vi "Ex-2 FPGA.vi"() -> ()   [LabVIEW 2014]
uses:
  <vilib>/rvi/Emulation/niFpgaGetClockAttributes.vi
  <vilib>/rvi/Emulation/niFpgaSctlEmulationGetInTimedLoop.vi
  <vilib>/rvi/Emulation/niFpgaEmulationReportErrorSimple.vi
  <vilib>/rvi/Emulation/niFpgaProcessEmulError.vi
  <vilib>/rvi/interface/RandomDataEmulation/niFpgaRandomDataHandleErrors.vi
  <vilib>/rvi/Emulation/niFpgaCriticalErrorInLSC.vi
  <vilib>/rvi/DataTransferAndStorage/Container/XNode/niFpgaContainer.xnode
  <vilib>/rvi/interface/RandomDataEmulation/nirviRandomDataFpgaReadWriteTemplate.vi
panel:
  in  "Data to Host":u64
  out "FPGA Error":errorcluster
  out "Finished":bool
  in  "stop":bool
  out "Module Underflow":bool
  out "Acq Loop Ticks":u32
  out "DMA FIFO Full":bool
  out "Chan Count":bool
  out "First Read":bool
  in  "Number of Channels":i32=4
  in  "Acquisition Type":enum16{"Finite Samples", "Continuous Samples"}(ring)
  in  "Samps per Chan [Finite]":i32=5120
  in  "Chan Scale Array":sgl[](array[numeric])=[0.0, 0.0, 0.0, 0.0, 0.0, 0.0, 0.0, 0.0, 0.0, 0.0, 0.0, 0.0, 0.0, 0.0, 0.0, 0.0, 0.0, 0.0, 0.0, 0.0, 0.0, 0.0, 0.0, 0.0, 0.0, 0.0, 0.0, 0.0, 0.0, 0.0, 0.0, 0.0, 0.0, 0.0, 0.0, 0.0, 0.0, 0.0, 0.0, 0.0]
  out "oclk mult":u32
  out "oclk div":u32
  out "oclk freq":u32
  in  "data rate (S/s)":u32
  # "Array size fixed at 40\nelements but may be \nexpanded if needed"
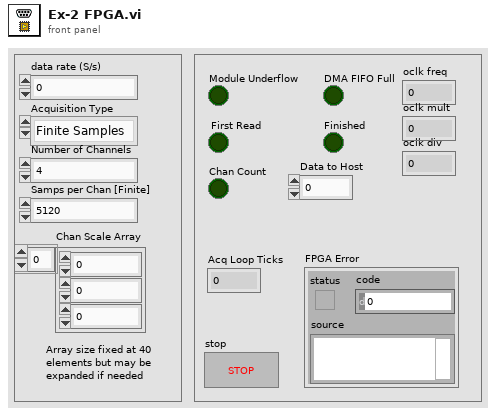
[diagram p1: front panel]
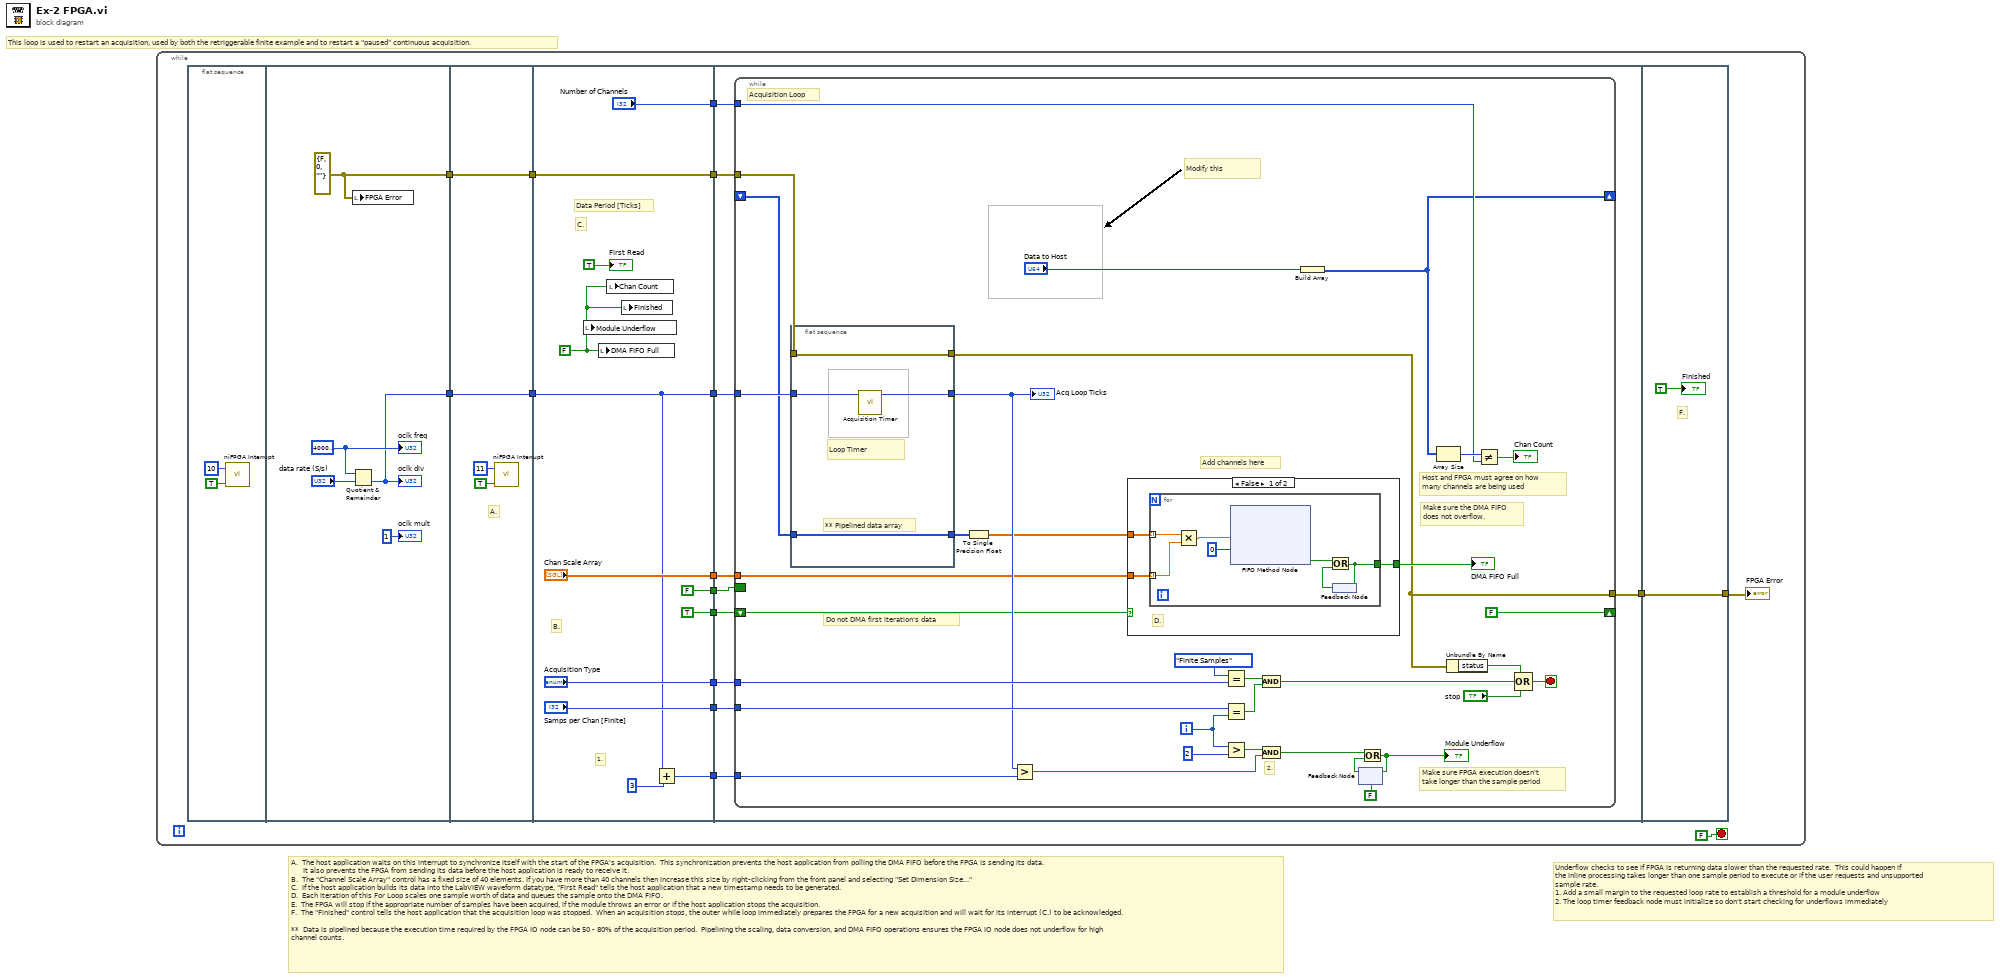
[diagram p0: block diagram]
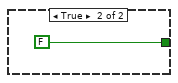
[diagram p2: hidden frame]
diagram:
  # "Underflow checks to see if FPGA is returning data slower than the requested rate.  This could happen if\nthe inline processing takes longer than one sample period to execute or if the user requests and unsupported\nsample rate.\n1. Add a small margin to the requested loop rate to establish a threshold for a module underflow \n2. The loop timer feedback node must initialize so don't start checking for underflows immediately"
  # "A.  The host application waits on this interrupt to synchronize itself with the start of the FPGA's acquisition.  This synchronization prevents the host application from polling the DMA FIFO before the FPGA is sending its data.\n      It also prevents the FPGA from sending its data before the host application is ready to receive it.\nB.  The \"Channel Scale Array\" control has a fixed size of 40 elements. If you have more than 40 channels then increase this size by right-clicking from the front panel and selecting \"Set Dimension Size...\"\nC.  If the host application builds its data into the LabVIEW waveform datatype, \"First Read\" tells the host application that a new timestamp needs to be generated.\nD.  Each iteration of this For Loop scales one sample worth of data and queues the sample onto the DMA FIFO.  \nE.  The FPGA will stop if the appropriate number of samples have been acquired, if the module throws an error or if the host application stops the acquisition.  \nF.  The \"Finished\" control tells the host application that the acquisition loop was stopped.  When an acquisition stops, the outer while loop immediately prepares the FPGA for a new acquisition and will wait for its interrupt (C.) to be acknowledged. \n\n**  Data is pipelined because the execution time required by the FPGA IO node can be 50 - 80% of the acquisition period.  Pipelining the scaling, data conversion, and DMA FIFO operations ensures the FPGA IO node does not underflow for high\nchannel counts."
  # "This loop is used to restart an acquisition, used by both the retriggerable finite example and to restart a \"paused\" continuous acquisition."
  n1 = while {
    stop <- FALSE stop-if-true
    n2 = flat-sequence {
      tunnel: [w20] -> w9
      tunnel: [w19] -> w5
      tunnel: w9 -> [w25]
      tunnel: [w25] -> w8
      tunnel: [w24] -> w6
      tunnel: w5 -> [w24]
      tunnel: ["Number of Channels"] -> w16
      tunnel: ["Chan Scale Array"] -> w15
      tunnel: ["Acquisition Type"] -> w14
      tunnel: ["Samps per Chan [Finite]"] -> w13
      tunnel: [w29] -> w12
      tunnel: [w33] -> w11
      tunnel: [TRUE] -> w10
      tunnel: w8 -> [w30]
      tunnel: [w30] -> w7
      tunnel: w6 -> [w29]
      tunnel: [FALSE] -> w4
      tunnel: w16 -> [w49]
      tunnel: w15 -> [w46]
      tunnel: w14 -> [w45]
      tunnel: w13 -> [w44]
      tunnel: w12 -> [w47]
      tunnel: w11 -> [w43]
      tunnel: w10 -> [w42]
      tunnel: w7 -> [w48]
      tunnel: w4 -> [w41]
      tunnel: [w40] -> w2
      tunnel: [w99] -> w1
      tunnel: w2 -> [w99]
      frame #0 {
        n3 = call <vilib>:"niFPGA Interrupt.vi"("Wait Until Cleared (F)"=TRUE ("Wait Until Cleared"), "IRQ Number (0)"=u8 10 ("IRQ Number")) -> ()  [unwired: 1 in]
      }
      frame #1 {
        w20 = errorcluster {"status"=FALSE, "code"=0, "source"=""} ("FPGA Error")
        w21 = u32 40000000 ("oclk freq")
        n4 = Quotient & Remainder(x=w21, y="data rate (S/s)") -> (floor(x/y)=w19:u32)  [unwired: 1 out]
        "oclk div" <- w19
        n5 = local write "FPGA Error"(w20) -> ()
        "oclk mult" <- u32 1 ("oclk mult")
        "oclk freq" <- w21
      }
      frame #2 {
        # "A."
        n6 = call <vilib>:"niFPGA Interrupt.vi"("Wait Until Cleared (F)"=TRUE ("Wait Until Cleared"), "IRQ Number (0)"=u8 11 ("IRQ Number")) -> ()  [unwired: 1 in]
      }
      frame #3 {
        w38 = FALSE ("Module Underflow")
        # "Data Period [Ticks]"
        # "1."
        # "C."
        # "B."
        n7 = local write "Module Underflow"(w38) -> ()
        n8 = local write "DMA FIFO Full"(w38) -> ()
        n9 = local write "Chan Count"(w38) -> ()
        n10 = local write "Finished"(w38) -> ()
        n11 = Add(x=w29, y=u32 3) -> (x+y=w33:u32)
        "First Read" <- TRUE ("First Read")
      }
      frame #4 {
        n12 = while {
          tunnel: w45 -> [w76]
          tunnel: w44 -> [w75]
          shift-right: [w55] -> _
          shift-left: _ -> [w67]
          tunnel: w49 -> [w77]
          tunnel: w48 -> [w69]
          tunnel: w47 -> [w74]
          tunnel: w43 -> [w70]
          tunnel: w46 -> [w66]
          shift-right: [FALSE] -> _
          shift-left: w42 -> [w65]
          border: w41 -> [_]
          tunnel: [w50] -> w40
          i -> [w63]
          stop <- w81 stop-if-true
          # "Modify this"
          # "Add channels here"
          # "2."
          # "Do not DMA first iteration's data"
          # "Host and FPGA must agree on how \nmany channels are being used"
          # "Acquisition Loop"
          # "Make sure the DMA FIFO\ndoes not overflow."
          # "Make sure FPGA execution doesn't\ntake longer than the sample period"
          n13 = flat-sequence {
            tunnel: w74 -> [w96]
            tunnel: [w98] -> w50
            tunnel: w69 -> [w98]
            tunnel: [w95] -> w68
            tunnel: [w97] -> w54
            tunnel: w67 -> [w97]
            frame #0 {
              # "Loop Timer"
              # "** Pipelined data array"
              n14 = call <vilib>:"Acquisition Timer.vi"("Loop Time (Ticks)"=w96) -> ("Actual Time (Ticks)"=w95:u32)  [unwired: 10 in]
            }
          }
          n15 = To Single Precision Float(number=w54) -> (single precision float=w53:sgl[])
          n16 = Greater?(x=w68, y=w70) -> (0:w73:bool)
          n17 = case shown="False" w65 {
            tunnel: [w86 FALSE] -> w80
            tunnel: w53 -> [w85 _]
            tunnel: w66 -> [w84 _]
            frame False {
              # "D."
              n18 = for {
                tunnel: [w92] -> w86
                tunnel: w85 -> [w91] mode=indexing
                tunnel: w84 -> [w87] mode=indexing
                n19 = Multiply(x=w91, y=w87) -> (x*y=w88:sgl)
                n20 = xnode ("FIFO Method Node")("Element"=w88, "Timeout"=0) -> ("Timed Out?"=w89:bool)  [unwired: 1 in, 1 out]
                n21 = feedback #1() -> (w93:bool)
                n22 = Or(x=w89, y=w93) -> (x .or. y?=w92:bool)
                n23 = feedback-in #1(w92) -> ()
              }
            }
            frame True {
            }
          }
          "DMA FIFO Full" <- w80
          n24 = Equal?(x=enum16{"Finite Samples", "Continuous Samples"}."Finite Samples" ("y"), y=w76) -> (x = y?=w58:bool)
          n25 = Equal?(x=w75, y=w63) -> (x = y?=w57:bool)
          n26 = Greater?(x=w63, y=2) -> (0:w72:bool)
          n27 = And(x=w58, y=w57) -> (x .and. y?=w56:bool)
          n28 = And(x=w72, y=w73) -> (x .and. y?=w60:bool)
          n29 = Build Array("Data to Host") -> (w55:u64[])
          n30 = feedback #2(FALSE) -> (w62:bool)
          n31 = Or(x=w60, y=w62) -> (x .or. y?=w59:bool)
          "Module Underflow" <- w59
          n32 = feedback-in #2(w59) -> ()
          n33 = Array Size(array=w55) -> (size(s)=w79:i32)
          n34 = Unbundle By Name(w50) -> ("status"=w51:bool)
          n35 = Not Equal?(x=w79, y=w77) -> (x != y?=→"Chan Count":bool)
          n36 = Compound Arithmetic op=OR(w51, w56, "stop") -> (w81:bool)
          "Acq Loop Ticks" <- w68
        }
      }
      frame #5 {
        # "F."
        "Finished" <- TRUE ("Finished")
      }
    }
    "FPGA Error" <- w1
  }
